vi "If statement else end index finder V1.vi"(10 "structure name":string, 11 "Auto Scripting array":T1) -> (2 "end index":i32, 3 "else index":i32)   [LabVIEW 2013]
uses:
  Autonmous Scripting array typedef.ctl
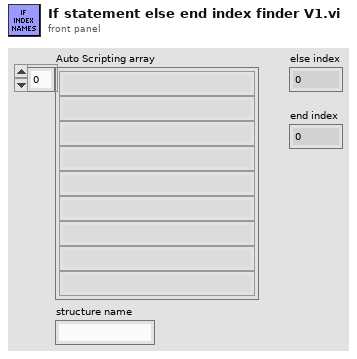
[diagram p1: front panel]
types:
  T1 = typedef "Autonmous Scripting array typedef.ctl" = string[]
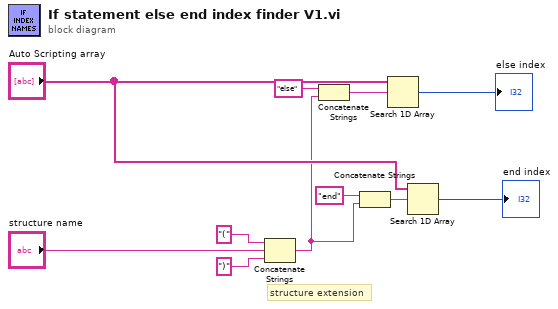
[diagram p0: block diagram]
diagram:
  # "structure extension"
  n1 = Concatenate Strings("(" ("string"), "structure name", ")" ("string")) -> (w2:string)
  n2 = Concatenate Strings("else" ("string"), w2) -> (w4:string)
  n3 = Concatenate Strings("end" ("string"), w2) -> (w1:string)
  n4 = Search 1D Array(1D array="Auto Scripting array", element=w4) -> (index of element=→"else index":i32)  [unwired: 1 in]
  n5 = Search 1D Array(1D array="Auto Scripting array", element=w1) -> (index of element=→"end index":i32)  [unwired: 1 in]
